vi "Build Description String.vi"(8 "error in (no error)":errorcluster, 11 "Mouse Macro in":refnum<class "Mouse Macro.lvclass">) -> (0 "error out":errorcluster, 2 "Description":string, 3 "Mouse Macro out":refnum<class "Mouse Macro.lvclass">)   [LabVIEW 2020, in "MacroAssert.lvlib" / "Mouse Macro.lvclass"]
doc: "Builds a string to describe what <B>Step</B> does."
uses:
  Mouse Macro.lvclass
  Mouse Macro.lvclass/Mouse Macro.ctl
  Macro Step/Macro Step.lvclass
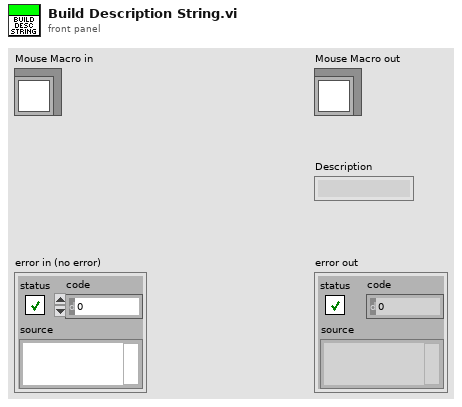
[diagram p1: front panel]
types:
  T1 = typedef "MacroAssert.lvlib/Step Type V3.ctl" = enum16{"Mouse Move", "Mouse Click", "Key Press", "Wait", "Mouse Down", "Mouse Up", "Key Down", "Key Up", "Test Assertion", "Maximize Window", "Restore Window", "Minimize Window", "Close Window", "Bring Window to Front", "Send Window to Back"}
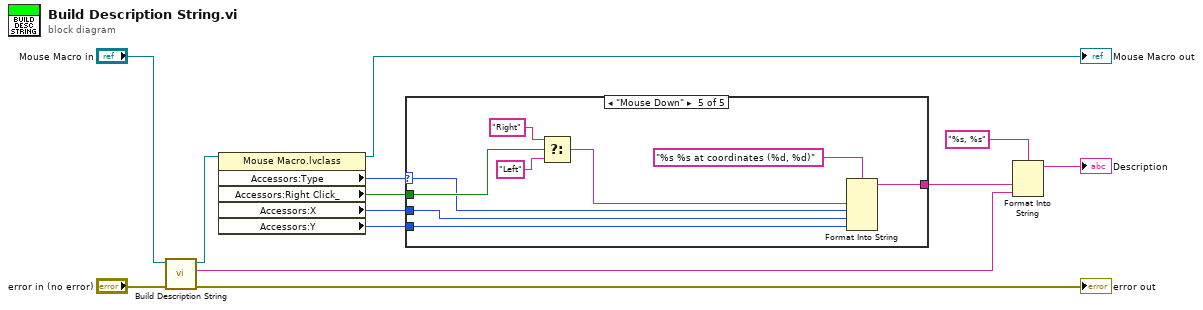
[diagram p0: block diagram]
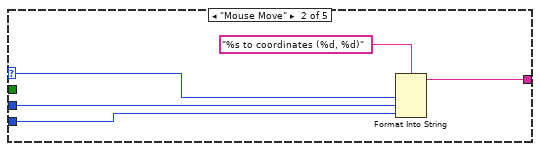
[diagram p3: hidden frame]
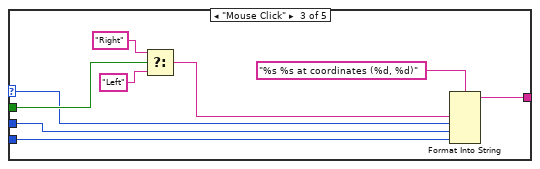
[diagram p4: hidden frame]
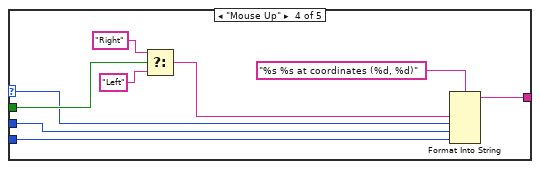
[diagram p5: hidden frame]
diagram:
  n1 = call-parent "Build Description String.vi"("error in (no error)"="error in (no error)", "Macro Step in"="Mouse Macro in") -> ("error out"=→"error out":errorcluster, "Description"=w1:string, "Macro Step out"=w5:refnum<class "Mouse Macro.lvclass">)  [unwired: 7 in]
  n2 = property class="Mouse Macro.lvclass"(reference=w5) -> (reference out=→"Mouse Macro out":refnum<class "Mouse Macro.lvclass">, "Accessors:Type"=w10:T1, "Accessors:Right Click_"=w9:bool, "Accessors:X"=w12:i32, "Accessors:Y"=w11:i32)  [unwired: 1 in, 1 out]
  n3 = case shown="\"Mouse Down\"" w10 {
    selector: w10 -> [_ w14 w19 w28 w37]
    tunnel: w9 -> [_ _ w21 w30 w39]
    tunnel: [_ w17 w26 w35 w44] -> w3
    tunnel: w12 -> [_ w16 w25 w34 w43]
    tunnel: w11 -> [_ w15 w24 w33 w42]
    frame Default {
    }
    frame "Mouse Move" {
      n4 = Format Into String(format string="%s to coordinates (%d, %d)", w14, w16, w15) -> (resulting string=w17:string)  [unwired: 2 in, 1 out]
    }
    frame "Mouse Click" {
      n5 = Select(t="Right", s=w21, f="Left") -> (s? t:f=w20:string)
      n6 = Format Into String(format string="%s %s at coordinates (%d, %d)", w20, w19, w25, w24) -> (resulting string=w26:string)  [unwired: 2 in, 1 out]
    }
    frame "Mouse Up" {
      n7 = Select(t="Right", s=w30, f="Left") -> (s? t:f=w29:string)
      n8 = Format Into String(format string="%s %s at coordinates (%d, %d)", w29, w28, w34, w33) -> (resulting string=w35:string)  [unwired: 2 in, 1 out]
    }
    frame "Mouse Down" {
      n9 = Select(t="Right", s=w39, f="Left") -> (s? t:f=w38:string)
      n10 = Format Into String(format string="%s %s at coordinates (%d, %d)", w38, w37, w43, w42) -> (resulting string=w44:string)  [unwired: 2 in, 1 out]
    }
  }
  n11 = Format Into String(format string="%s, %s", w3, w1) -> (resulting string=→"Description":string)  [unwired: 2 in, 1 out]
